vi "Set-visibility.vi"(8 "error in (no error)":errorcluster, 9 "Visibility":bool, 10 "Pane":T1, 11 "Panes in":T2) -> (0 "error out":errorcluster, 3 "Panes out":T2)   [LabVIEW 2013, in "MaterialCharacterization.lvlib" / "MC-UI.lvclass"]
uses:
  MC-UI.lvclass
  Panes-reference.ctl
  Pane-names.ctl
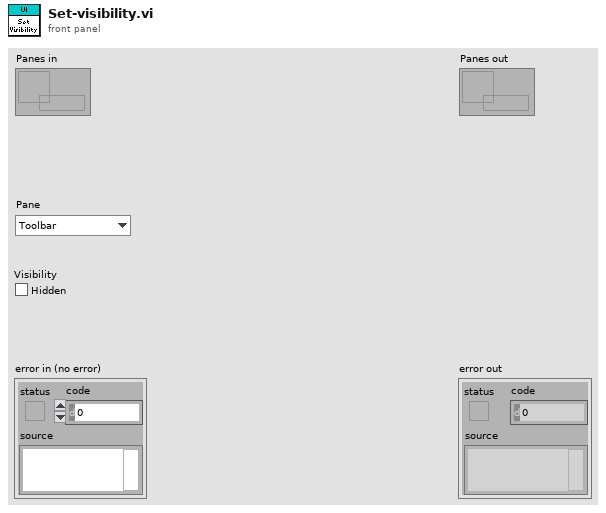
[diagram p1: front panel]
types:
  T1 = typedef "MaterialCharacterization.lvlib/MC-UI.lvclass/Pane-names.ctl" = enum16{"Toolbar", "Help bar", "Toolbar lower border", "Center panel", "Main panel", "Settings panel", "Status bar upper border", "General state bar", "Information bar"}
  T2 = typedef "MaterialCharacterization.lvlib/MC-UI.lvclass/Panes-reference.ctl" = refnum<data-value>
  T3 = typedef "MaterialCharacterization.lvlib/MC-UI.lvclass/Pane-settings.ctl" = cluster{"Pane-name":T1, "Startup status":bool, "Current status":bool, "Splitters":T4[], "Pane-reference":refnum<vi>}
  T4 = typedef "MaterialCharacterization.lvlib/MC-UI.lvclass/Splitter-settings.ctl" = cluster{"Splitter-name":T5, "Position shown":i32, "Position hidden":i32, "Splitter reference":refnum<vi>}
  T5 = typedef "MaterialCharacterization.lvlib/MC-UI.lvclass/Splitter-names.ctl" = enum16{"Upper toolbar splitter", "Help bar splitter", "Lower toolbar splitter", "Upper status bar splitter", "Lower status bar splitter", "Left status bar splitter", "Settings splitter"}
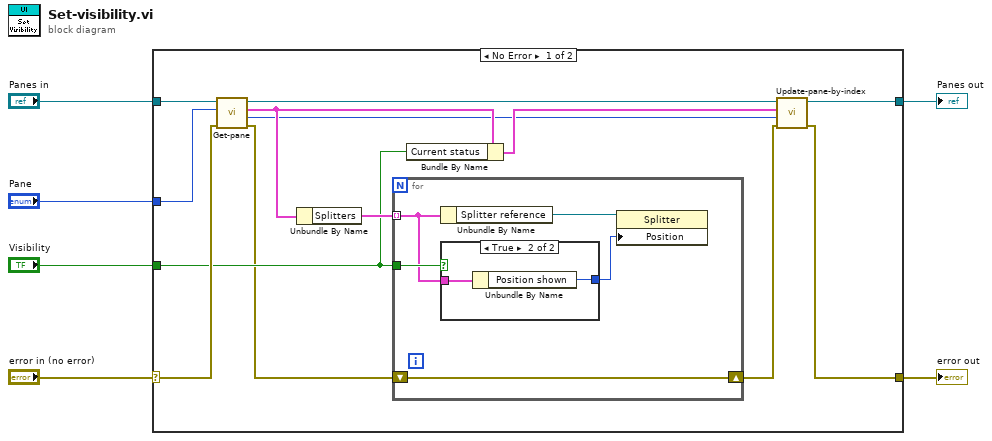
[diagram p0: block diagram]
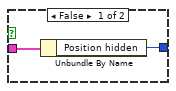
[diagram p2: hidden frame]
diagram:
  n1 = case shown="No Error" "error in (no error)" {
    selector: "error in (no error)" -> [w17 w29]
    tunnel: [w10 w29] -> w5
    tunnel: [w9 w30] -> w3
    tunnel: "Panes in" -> [w19 w30]
    tunnel: "Pane" -> [w18 _]
    tunnel: "Visibility" -> [w14 _]
    frame No Error {
      n2 = call "Get-pane.vi"("error in (no error)"=w17, "Pane"=w18, "Panes in"=w19) -> ("error out"=w8:errorcluster, "Index"=w11:i32, "Pane"=w15:T3, "Panes out"=w13:T2)  [unwired: 5 in]
      n3 = Unbundle By Name(w15) -> ("Splitters"=w16:T4[])
      n4 = for {
        tunnel: w14 -> [w24]
        tunnel: w16 -> [w23] mode=indexing
        shift-right: [w20] -> w7
        shift-left: w8 -> [w20]
        n5 = Unbundle By Name(w23) -> ("Splitter reference"=w22:refnum<vi>)
        n6 = case shown="True" w24 {
          tunnel: w23 -> [w26 w28]
          tunnel: [w25 w27] -> w21
          frame False {
            n7 = Unbundle By Name(w26) -> ("Position hidden"=w25:i32)
          }
          frame True {
            n8 = Unbundle By Name(w28) -> ("Position shown"=w27:i32)
          }
        }
        n9 = property class="Splitter"(reference=w22, "Position"=w21) -> ()  [unwired: 1 in, 2 out]
      }
      n10 = Bundle By Name(cluster=w15, "Current status"=w14) -> (w12:T3)
      n11 = call "Update-pane-by-index.vi"("error in (no error)"=w7, "Pane index"=w11, "Pane"=w12, "Panes in"=w13) -> ("error out"=w10:errorcluster, "Panes out"=w9:T2)  [unwired: 6 in]
    }
    frame Error {
    }
  }
  "error out" <- w5
  "Panes out" <- w3
